vi "FRCts20_Backend_Dyn_Unload_VIs.vi"(8 "error in":errorcluster, 11 "VI Names and Refnums":T1[](array[typedef])) -> (0 "error out":errorcluster, 3 "VI Names":path[](array[path]))   [LabVIEW 2013, in "FRCts20_Backend_Engine.lvlib"]
uses:
  FRCts20_Backend_Engine.lvlib
  FRCts20_Backend_Dyn_Refnums.ctl
  INI_Accessor/FRCts20_Backend_INI Controller.lvclass
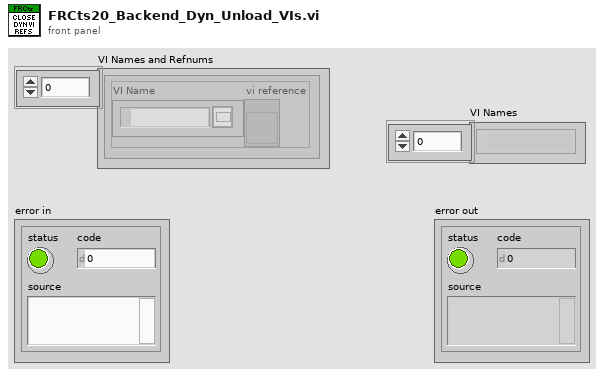
[diagram p1: front panel]
types:
  T1 = typedef "FRCts20_Backend_Engine.lvlib/FRCts20_Backend_Dyn_Refnums.ctl" = cluster{"VI Name":path, "vi reference":refnum<vi>}
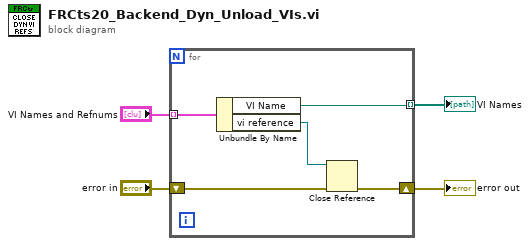
[diagram p0: block diagram]
diagram:
  n1 = for {
    shift-right: [w5] -> w3
    shift-left: "error in" -> [w7]
    tunnel: "VI Names and Refnums" -> [w9] mode=indexing
    tunnel: [w8] -> w1 mode=indexing
    n2 = Unbundle By Name(w9) -> ("VI Name"=w8:path, "vi reference"=w6:refnum<vi>)
    n3 = Close Reference(reference=w6, error in (no error)=w7) -> (error out=w5:errorcluster)
  }
  "VI Names" <- w1
  "error out" <- w3
